vi "LIN Slave Get Data.vi"(10 "LINIndex":u8, 11 "DevHandle":i32) -> (2 "function return":i32, 3 "pLINMsg":T1)   [LabVIEW 2010, in "USB2XXX.lvlib"]
doc: "int WINAPI LIN_SlaveGetData(int DevHandle,unsigned char LINIndex,LIN_MSG *pLINMsg);"
uses:
  USB2XXX.lvlib
  USB2XXX.dll
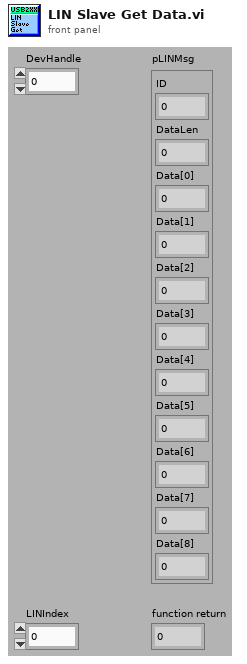
[diagram p1: front panel]
types:
  T1 = cluster{"ID":u8, "DataLen":u8, "Data[0]":u8, "Data[1]":u8, "Data[2]":u8, "Data[3]":u8, "Data[4]":u8, "Data[5]":u8, "Data[6]":u8, "Data[7]":u8, "Data[8]":u8}
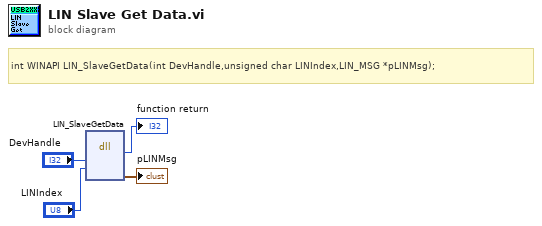
[diagram p0: block diagram]
diagram:
  # "int WINAPI LIN_SlaveGetData(int DevHandle,unsigned char LINIndex,LIN_MSG *pLINMsg);"
  n1 = dll-call lib="F:/OtherWork/STM32/USB2XXX_Example/trunk/Labview/PublicFiles/USB2XXX.*" fn="LIN_SlaveGetData"("DevHandle"="DevHandle", "LINIndex"="LINIndex") -> (→"function return":i32, "pLINMsg"=→"pLINMsg":T1)  [unwired: 6 in, 2 out]
